vi "Recieve I32 Data.vi"(8 "error in (no error)":errorcluster, 9 "bytes per sample":i32=12, 10 "Samples per read":i32=1024, 11 "RP Communicator in":refnum<class "RP Communicator.lvclass">) -> (0 "error out":errorcluster, 2 "Data out":i32[](array[numeric]), 3 "RP Communicator out":refnum<class "RP Communicator.lvclass">)   [LabVIEW 2019, in "RP Communicator.lvclass"]
uses:
  RP Communicator.lvclass
  RP Read RX FIFO Fast TCP.vi
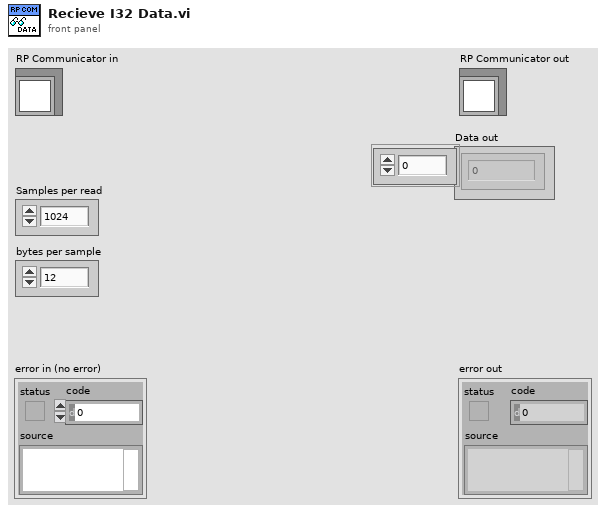
[diagram p1: front panel]
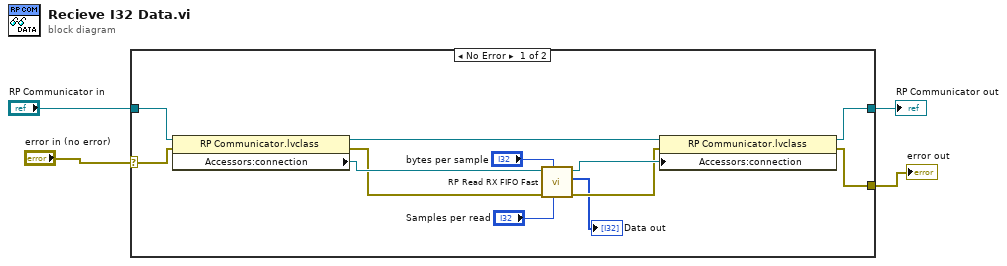
[diagram p0: block diagram]
diagram:
  n1 = case shown="No Error" "error in (no error)" {
    selector: "error in (no error)" -> [w8 w18]
    tunnel: [w7 w18] -> w3
    tunnel: [w6 w17] -> w1
    tunnel: "RP Communicator in" -> [w16 w17]
    frame No Error {
      n2 = property class="RP Communicator.lvclass"(reference=w16, error in=w8) -> (reference out=w15:refnum<class "RP Communicator.lvclass">, error out=w10:errorcluster, "Accessors:connection"=w14:refnum<k5>)
      n3 = call-poly "RP Read RX FIFO Fast.vi"("Samples per read"="Samples per read", "bytes per sample"="bytes per sample", "Error In"=w10, "connection ID"=w14) -> ("Error Out"=w9:errorcluster, "FIFO out"=→"Data out":i32[], "connection ID out"=w13:refnum<k5>)  [unwired: 5 in]
      n4 = property class="RP Communicator.lvclass"(reference=w15, error in=w9, "Accessors:connection"=w13) -> (reference out=w6:refnum<class "RP Communicator.lvclass">, error out=w7:errorcluster)
    }
    frame Error {
    }
  }
  "error out" <- w3
  "RP Communicator out" <- w1
